vi "AlliGator Update Decay Fit Parameter Map Palette.vi"(8 "error in (no error)":errorcluster, 10 "Image Display Palette Information":T2 {"Palette Type" items=["Grayscale", "Binary", "Gradient", "Rainbow", "Temperature", "User Defined", "Binary 16 Bit", "Gradient 16 Bit", "Rainbow 16 Bit", "Temperature 16 Bit", "User Defined 16 Bit"]}, 11 "Decay Fit Map Ctrl Refums":T1) -> (0 "error out":errorcluster)   [LabVIEW 2021, in "AlliGator Decay Fit Parameter Map.lvlib"]
doc: "Updates the color palette of the <B>Decay Fit Parameter Map</B> image."
uses:
  AlliGator Decay Fit Parameter Map.lvlib
  Palette/Image Palette Information.ctl
  Image/Image Display Palette Type.ctl
  AlliGator Decay Fit Map Control Refnums.ctl
  Fits/IRF(X)PSED/Decay Fit Parameters & Derived Quantities List v2.ctl
  Image/Image.lvlib
  Palette/Palette.lvlib
  Fits/Fits.lvlib
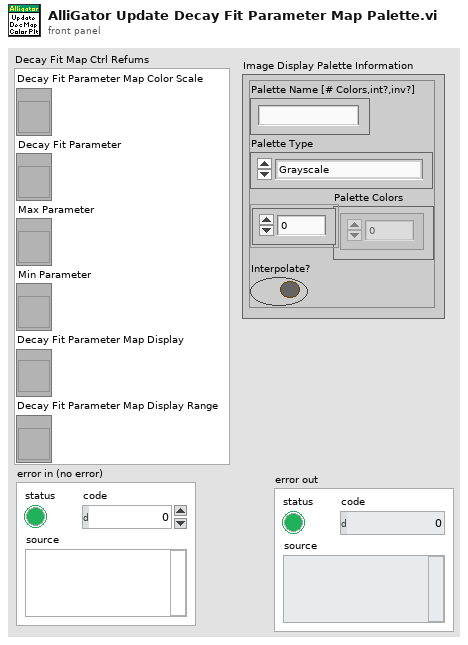
[diagram p1: front panel]
types:
  T1 = typedef "AlliGator Decay Fit Parameter Map.lvlib/AlliGator Decay Fit Map Control Refnums.ctl" = cluster{"Decay Fit Parameter Map Color Scale":refnum<vi>, "Decay Fit Parameter":refnum<vi>, "Max Parameter":refnum<vi>, "Min Parameter":refnum<vi>, "Decay Fit Parameter Map Display":refnum<vi>, "Decay Fit Parameter Map Display Range":refnum<vi>}
  T2 = typedef "Palette.lvlib/Image Palette Information.ctl" = cluster{"Palette Name [# Colors,int?,inv?]":string, "Palette Type":T3, "Palette Colors":u32[], "Interpolate?":bool}
  T3 = typedef "Image.lvlib/Image Display Palette Type.ctl" = u32
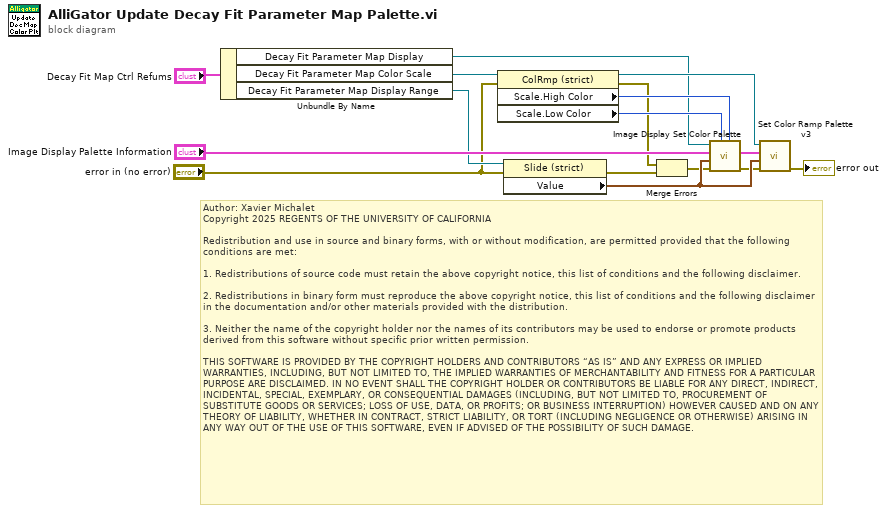
[diagram p0: block diagram]
diagram:
  # "Author: Xavier Michalet\nCopyright 2025 REGENTS OF THE UNIVERSITY OF CALIFORNIA\n\nRedistribution and use in source and binary forms, with or without modification, are permitted provided that the following conditions are met:\n\n1. Redistributions of source code must retain the above copyright notice, this list of conditions and the following disclaimer.\n\n2. Redistributions in binary form must reproduce the above copyright notice, this list of conditions and the following disclaimer in the documentation and/or other materials provided with the distribution.\n\n3. Neither the name of the copyright holder nor the names of its contributors may be used to endorse or promote products derived from this software without specific prior written permission.\n\nTHIS SOFTWARE IS PROVIDED BY THE COPYRIGHT HOLDERS AND CONTRIBUTORS “AS IS” AND ANY EXPRESS OR IMPLIED WARRANTIES, INCLUDING, BUT NOT LIMITED TO, THE IMPLIED WARRANTIES OF MERCHANTABILITY AND FITNESS FOR A PARTICULAR PURPOSE ARE DISCLAIMED. IN NO EVENT SHALL THE COPYRIGHT HOLDER OR CONTRIBUTORS BE LIABLE FOR ANY DIRECT, INDIRECT, INCIDENTAL, SPECIAL, EXEMPLARY, OR CONSEQUENTIAL DAMAGES (INCLUDING, BUT NOT LIMITED TO, PROCUREMENT OF SUBSTITUTE GOODS OR SERVICES; LOSS OF USE, DATA, OR PROFITS; OR BUSINESS INTERRUPTION) HOWEVER CAUSED AND ON ANY THEORY OF LIABILITY, WHETHER IN CONTRACT, STRICT LIABILITY, OR TORT (INCLUDING NEGLIGENCE OR OTHERWISE) ARISING IN ANY WAY OUT OF THE USE OF THIS SOFTWARE, EVEN IF ADVISED OF THE POSSIBILITY OF SUCH DAMAGE."
  n1 = Unbundle By Name("Decay Fit Map Ctrl Refums") -> ("Decay Fit Parameter Map Display"=w1:refnum<vi>, "Decay Fit Parameter Map Color Scale"=w8:refnum<vi>, "Decay Fit Parameter Map Display Range"=w6:refnum<vi>)
  n2 = property on="Property Node" class="ColRmp (strict)"(reference=w8, error in="error in (no error)") -> (reference out=w7:refnum<vi>, error out=w4:errorcluster, "Scale.High Color"=w11:u32, "Scale.Low Color"=w15:u32)
  n3 = property on="Property Node" class="Slide (strict)"(reference=w6, error in="error in (no error)") -> (error out=w2:errorcluster, "Value"=w13:cluster{dbl, dbl})  [unwired: 1 out]
  n4 = Merge Errors(w4, w2) -> (w3:errorcluster)
  n5 = call "Image Display Set Color Palette.vi"("Image High Color"=w11, "Image Low Color"=w15, "Error In"=w3, "Image Display Range"=w13, "Image Display Palette Information"="Image Display Palette Information", "Display Image Control Refnum"=w1) -> ("Error Out"=w12:errorcluster)  [unwired: 5 in]
  n6 = call "Set Color Ramp Palette v3.vi"("error in (no error)"=w12, "Image Display Range"=w13, "Image Display Palette Information"="Image Display Palette Information", "ColorRamp in"=w7) -> ("Error Out"=→"error out":errorcluster)  [unwired: 5 in, 2 out]
